vi "Modtag_billede_og_split.vi"() -> ()   [LabVIEW 2018]
uses:
  <vilib>/myRIO/Instrument Drivers/Onboard IO/UART/typedef/VISA Configuration.ctl
  <vilib>/Instr/_visa.llb/VISA Configure Serial Port (Instr).vi
  <vilib>/myRIO/Express VI/Onboard IO/UART/UART Express VI.xnode
  <vilib>/myRIO/Instrument Drivers/Onboard IO/UART/UART.lvlib
panel:
  out "Intensity Graph 4":u8[][](graph)
  in  "stop":bool
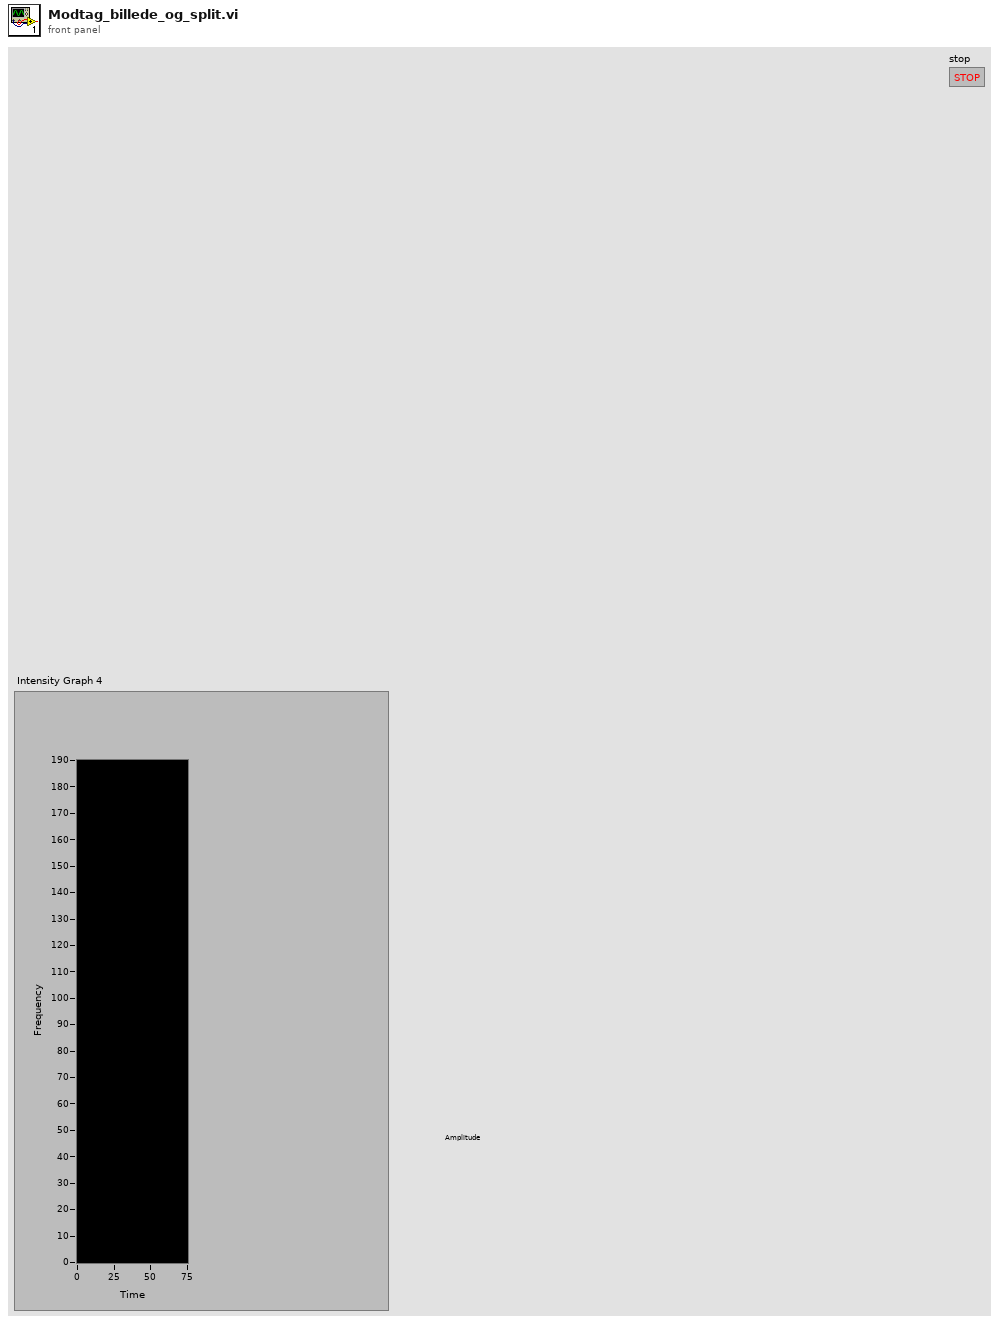
[diagram p1: front panel]
types:
  T1 = typedef "UART.lvlib/VISA Configuration.ctl" = cluster{"baud rate (9600)":u32, "data bits (8)":u16, "parity (0:none)":enum16{"None", "Odd", "Even", "Mark", "Space"}, "stop bits (10: 1 bit)":u16, "flow control (0:none)":u16, "termination char\n(0xA = '\\n' = LF) ":u8, "Enable Termination\nChar (T)":bool, "timeout (10sec)":u32}
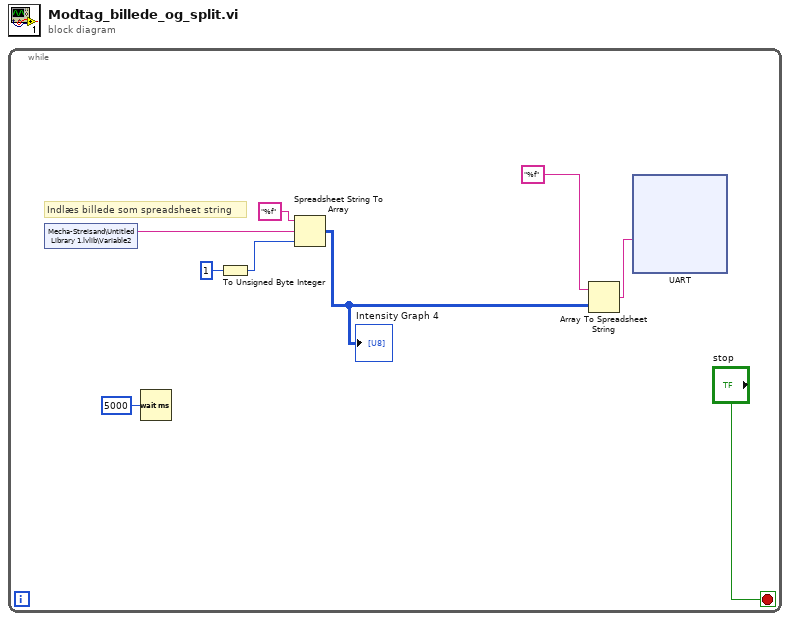
[diagram p0: block diagram]
diagram:
  n1 = while {
    stop <- "stop" stop-if-true
    # "Indlæs billede som spreadsheet string"
    n2 = shared-variable "Mecha-Streisand\\Untitled Library 1.lvlib\\Variable2"() -> (w7:string)  [unwired: 1 in, 1 out]
    n3 = Wait (ms)(milliseconds to wait=u32 5000) -> ()  [unwired: 1 out]
    n4 = To Unsigned Byte Integer(number=u8 1) -> (unsigned 8bit integer=w9:u8)
    n5 = Spreadsheet String To Array(format string="%f", spreadsheet string=w7, array type (2D Dbl)=w9) -> (array=w1:u8[][])  [unwired: 1 in]
    "Intensity Graph 4" <- w1
    n6 = Array To Spreadsheet String(array=w1, 3:"%f" ("format string")) -> (spreadsheet string=w3:string)  [unwired: 1 in]
    n7 = xnode "UART"("Characters to Write"=w3) -> ()  [unwired: 1 in, 2 out]
  }
